vi "clog2.vi"(11 "Number":u32 format="%.0f (%b)") -> (3 "clog2":i32)   [LabVIEW 2016]
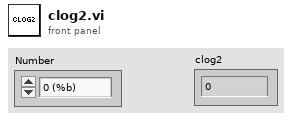
[diagram p1: front panel]
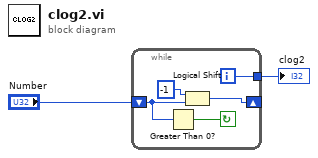
[diagram p0: block diagram]
diagram:
  n1 = while {
    tunnel: [w5] -> w1
    shift-right: [w3] -> _
    shift-left: "Number" -> [w4]
    i -> [w5]
    stop <- w6 continue-if-true
    n2 = Greater Than 0?(x=w4) -> (x > 0?=w6:bool)
    n3 = Logical Shift(y=i16 -1, x=w4) -> (x << y=w3:u32)
  }
  "clog2" <- w1
